vi "Charger_Telem with Retries.vi"(8 "error in":errorcluster, 9 "Charger Inputs":T4 {"setpoint" min=0.0 max=20000.0 step=100.0; "position" min=0 max=5 step=1}, 10 "MICS Input":T2, 11 "MICS Dongle Address":refnum<visa-resource-name>) -> (0 "error out":errorcluster, 2 "Output":T3)   [LabVIEW 2020]
uses:
  Charger_Input Control.ctl
  Telemetry/Typedef Command List.ctl
  Charging/Charging_MICS Retry Count.vi
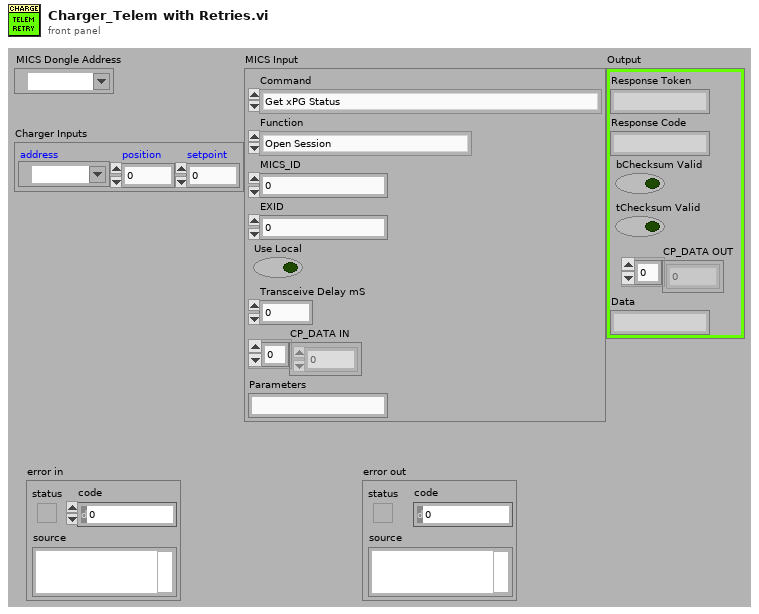
[diagram p1: front panel]
types:
  T1 = typedef "Typedef Command List.ctl" = enum16{"Get xPG Status", "xPG Stimulation", "Select Program", "Increment Program Amplitude", "Decrement Program Amplitude", "Get PoP Constants", "Get PPC Constants", "Get Program Names", "Set Pulse Amplitude", "Increment Pulse Amplitude", "Decrement Pulse Amplitude", "Get Pulse Widths", "Set Pulse Widths", "Increment Pulse Width", "Decrement Pulse Width", "Get Program Frequency", "Set Program Frequency", "Increment Program Frequency", "Decrement Program Frequency", "Inject Event", "Charging Control", "Get xPG Identity", "Set xPG Identity", "Restore Program Defaults", "Get Program Definition", "Set Program Definition", "Get Program Constants", "Set Program Constants", "Get Configurable Device Parameters", "Set Configurable Device Parameters", "Get Pulse Constants", "Set Pulse Constants", "Get Lead Limits", "Set Lead Limits", "Get Channel Calibrations", "Set Channel Calibrations", "<reserved 2>", "<reserved 3>", "<reserved 4>", "<reserved 5>", "<reserved 6>", "<reserved 7>", "Get Stim Asic HV Calibrations", "Set Stim Asic HV Calibrations", "<reserved 8>", "<reserved 9>", "Get CP Data", "Set CP Data", "Clear Log", "Read Log", "Append Log", "Get Patient Program Runtime", "Set Patient Program Runtime", "Impedance Measurement", "Enter Storage Mode", "Echo Short", "Echo Long", "Get General Calibration", "Set General Calibration", "Get Trim List", "Set Trim List", "Get Counter", "Set Counter", "Get Test Stimulation", "Set Test Stimulation", "Get Titration Stimulation", "Set Titration Stimulation", "Get Ramp Time", "Set Ramp Time", "Get VBAT", "Set Software Description Block", "Get Software Description Block", "Write Memory", "Read Memory", "Reset xPG", "Erase Flash Block", "Write Vectors", "Read Vectors", "Diagnostic Data", "Set Background Impedance", "Get Background Impedence ", "Set Test Waveform", "Calibrate Channel", "Get Log Range", "Reserved 0x55", "Reserved 0x56", "MICS Options", "Pair PPC", "Pair POP", "Stop Bootloader", "Tune MICS", "MICS Diagnostics", "Undefined"}
  T2 = cluster{"Command":T1, "Function":enum16{"Open Session", "Close Session", "Downlink Only", "Uplink Only", "Transceive (DN -> UP)"}, "MICS_ID":u32, "EXID":u32, "Use Local":bool, "Transceive Delay mS":dbl, "CP_DATA IN":u8[], "Parameters":string}
  T3 = cluster{"Response Token":string, "Response Code":string, "bChecksum Valid":bool, "tChecksum Valid":bool, "CP_DATA OUT":u8[], "Data":string}
  T4 = typedef "Charger_Input Control.ctl" = cluster{"address":refnum<visa-resource-name>, "position":i32, "setpoint":dbl}
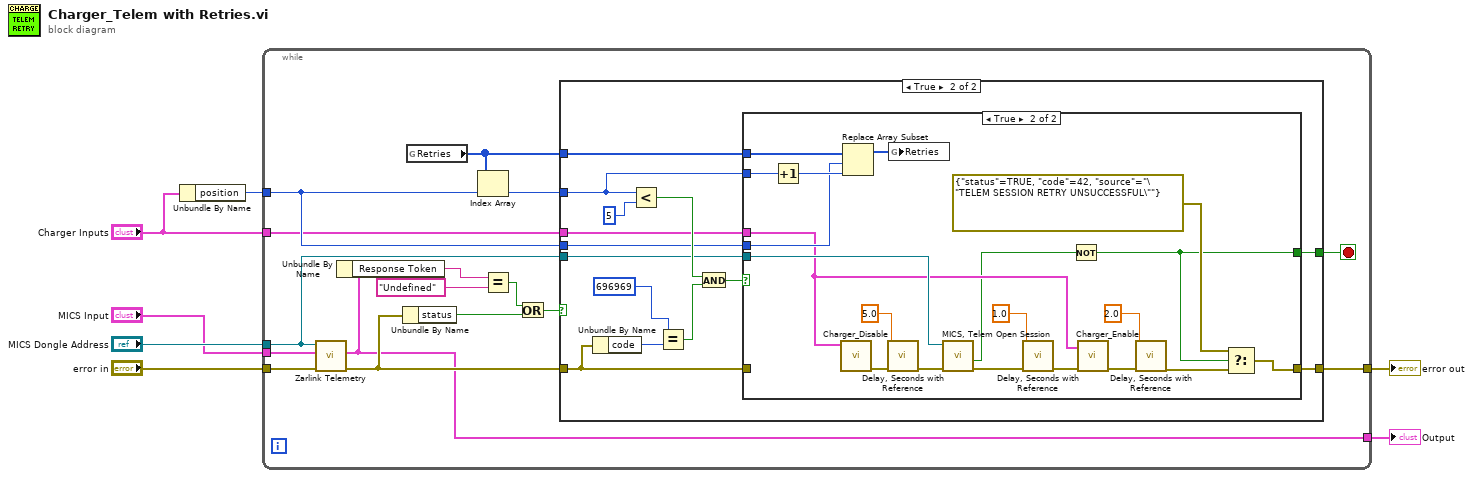
[diagram p0: block diagram]
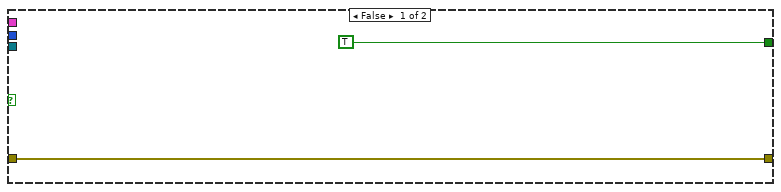
[diagram p2: hidden frame]
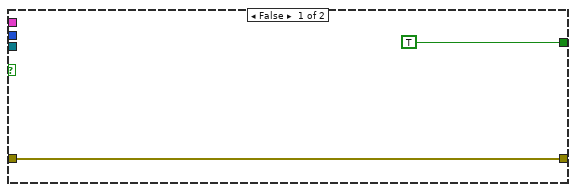
[diagram p3: hidden frame]
diagram:
  n1 = Unbundle By Name("Charger Inputs") -> ("position"=w1:i32)
  n2 = while {
    tunnel: "MICS Input" -> [w23]
    tunnel: [w11] -> w4
    tunnel: "error in" -> [w22]
    tunnel: "MICS Dongle Address" -> [w16]
    tunnel: [w21] -> w7
    tunnel: w1 -> [w18]
    tunnel: "Charger Inputs" -> [w15]
    stop <- w17 stop-if-true
    n3 = call "Zarlink Telemetry.vi"("error in (no error)"=w22, "Input"=w23, "MICS Dongle Address"=w16) -> ("error out"=w13:errorcluster, "Output"=w11:T3)  [unwired: 6 in, 1 out]
    n4 = Unbundle By Name(w11) -> ("Response Token"=w10:string)
    n5 = Unbundle By Name(w13) -> ("status"=w12:bool)
    n6 = global read "Charging_MICS Retry Count.vi" "Retries"() -> (w19:u8[])
    n7 = Index Array(array=w19, index=w18) -> (element=w20:u8)
    n8 = Equal?(x=w10, y="Undefined") -> (x = y?=w8:bool)
    n9 = Or(x=w8, y=w12) -> (x .or. y?=w14:bool)
    n10 = case shown="True" w14 {
      tunnel: [w24 w37] -> w21
      tunnel: w20 -> [_ w31]
      tunnel: w19 -> [_ w32]
      tunnel: w18 -> [_ w30]
      tunnel: [TRUE w29] -> w17
      tunnel: w16 -> [_ w28]
      tunnel: w15 -> [_ w27]
      tunnel: w13 -> [w24 w26]
      frame False {
      }
      frame True {
        n11 = Unbundle By Name(w26) -> ("code"=w39:i32)
        n12 = Less?(x=w31, y=u8 5) -> (x < y?=w34:bool)
        n13 = Equal?(x=696969, y=w39) -> (x = y?=w35:bool)
        n14 = And(x=w34, y=w35) -> (x .and. y?=w33:bool)
        n15 = case shown="True" w33 {
          tunnel: w26 -> [w41 _]
          tunnel: [w41 w42] -> w37
          tunnel: w32 -> [_ w61]
          tunnel: w31 -> [_ w60]
          tunnel: w30 -> [_ w58]
          tunnel: [TRUE w43] -> w29
          tunnel: w28 -> [_ w56]
          tunnel: w27 -> [_ w52]
          frame False {
          }
          frame True {
            n16 = Increment(x=w60) -> (x+1=w59:u8)
            n17 = call "Charger_Disable.vi"("Charger"=w52) -> ("error out"=w55:errorcluster)  [unwired: 8 in]
            n18 = Replace Array Subset(array=w61, new element=w59, index=w58) -> (w57:u8[])
            n19 = call "Delay, Seconds with Reference.vi"("error in"=w55, "delay"=dbl[unit] 5.0) -> ("error out"=w54:errorcluster)  [unwired: 4 in, 2 out]
            n20 = global write "Charging_MICS Retry Count.vi" "Retries"(w57) -> ()
            n21 = call "MICS, Telem Open Session.vi"("error in"=w54, "VISA resource"=w56) -> ("error out"=w47:errorcluster, "in_session"=w46:bool)  [unwired: 7 in, 1 out]
            n22 = call "Delay, Seconds with Reference.vi"("error in"=w47, "delay"=dbl[unit] 1.0) -> ("error out"=w53:errorcluster)  [unwired: 4 in, 2 out]
            n23 = Not(x=w46) -> (.not. x?=w43:bool)
            n24 = call "Charger_Enable.vi"("error in"=w53, "Charger"=w52) -> ("error out"=w49:errorcluster)  [unwired: 7 in]
            n25 = call "Delay, Seconds with Reference.vi"("error in"=w49, "delay"=dbl[unit] 2.0) -> ("error out"=w45:errorcluster)  [unwired: 4 in, 2 out]
            n26 = Select(t=errorcluster {"status"=TRUE, "code"=42, "source"="\"TELEM SESSION RETRY UNSUCCESSFUL\""} ("error out"), s=w43, f=w45) -> (s? t:f=w42:errorcluster)
          }
        }
      }
    }
  }
  "error out" <- w7
  "Output" <- w4
